vi "Untitled 1.vi"() -> ()   [LabVIEW 2015]
uses:
  <vilib>/Utility/miscctls.llb/LVRowAndColumnTypeDef.ctl
panel:
  in  "Active Cell:Active Cell":T1
  in  "Feature List":i32(listbox) caption="Steps List"
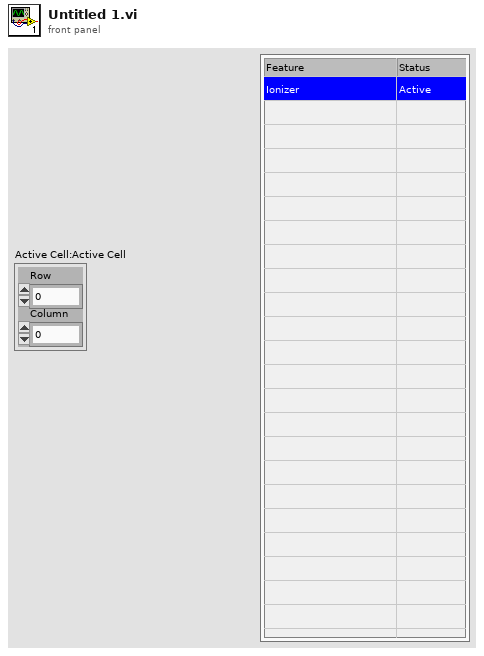
[diagram p1: front panel]
types:
  T1 = typedef "LVRowAndColumnTypeDef.ctl" = cluster{"Row":i32, "Column":i32}
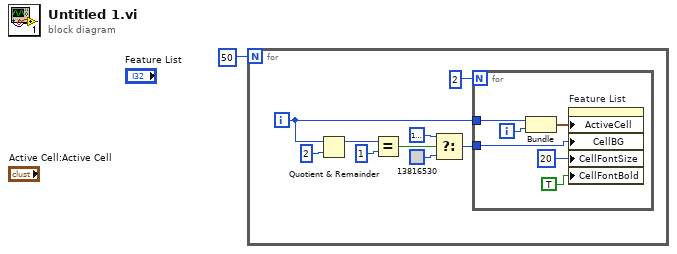
[diagram p0: block diagram]
diagram:
  n1 = for {
    N: 50 -> [_]
    i -> [w9]
    n2 = Quotient & Remainder(x=w9, y=2) -> (x-y*floor(x/y)=w7:i32)  [unwired: 1 out]
    n3 = Equal?(x=w7, y=1) -> (x = y?=w5:bool)
    n4 = Select(t=u32 16777225 ("Color Box"), s=w5, f=u32 13816530 ("Color Box")) -> (s? t:f=w2:u32)
    n5 = for {
      N: 2 -> [_]
      tunnel: w9 -> [w16]
      tunnel: w2 -> [w13]
      i -> [w15]
      n6 = Bundle(w16, w15) -> (w14:cluster{i32, i32})  [unwired: 1 in]
      n7 = property on="Feature List" class="MCListbox (strict)"("ActiveCell"=w14, "CellBG"=w13, "CellFontSize"=u32 20 ("Active Cell:Cell Font:Size"), "CellFontBold"=TRUE ("Active Cell:Cell Font:Bold")) -> ()  [unwired: 2 in, 2 out]
    }
  }
